vi "ORS_Samples_per_Line.vi"(2 "SPLL RF Clocks/Sweep":dbl=2560.0, 3 "Buffer_factor":i32=1, 4 "f_FDML":dbl=100000.0, 5 "General state cluster":T5={"millisecond timer value"=0, "PreviewSetNumberOfLines"=512, "Data source"=enum."AlazarTec", "DLL path"=path "M:/Optores_MHzImaging/WWImgDLL/wwimg-x86_64.dll", "n_threads"=1, "selected A-scan"={[], "cut_data"=[]}, "FDML freq"=100000.0, "Sample Rate"=500000000.0, "n_channel"=1, "Peak samp pos\n1mm (Michels)"=143, "Buffer factor"=1, "At9462Acq"={"sample_rate"=0, "clock source"=1}, "At9462Trig"={"trig_source"=enum."Ext", "trig_slope"=0, "trig_level"=0, "trig_timeout_ms"=0}, "At9462Ch1"={"coupling"=0, "range"=0, "impedance"=0}, "At9462Ch2"={"coupling"=0, "range"=0, "impedance"=0}, "At9462 # samples"=2560, "image height (crop)"=512, "B scan offset (sps)"=0.0, "window"=0, "OCT data dir"=path "", "2d file name"="", "3d file name"="", "# lines 2d"=1024, "Description"="", "Various parameters"="", "# linesPreview/jpg"=512, "# lines 3d"=512, "Y center 3d"=0.0, "Y span 3d"=0.0, "Galvo params only for file storage"={"n_lines"=400, "n_frames"=100, "force to zero"=TRUE, "Triggers_per_sweep"=1.0, "X center"=0.0, "X span"=5.6, "Y center"=0.0, "Y span"=0.0, "flyb.lines"=100, "n_triggers"=1, "mode"=3, "offset"=0.0, "galvo phase"=-15, "span factor"=0.0, "Custom trig."={"n_frames to c. trig"=0, "custom trig length (frames)"=0, "n_frames between c. trig"=0, "n_c. trig"=0}, "frames_per_pos"=5, "n_dataset"=1, "flyback fr"=0}, "Per Channel Params"=[{"AcqCursorList"=[{"Name"="img start", "Color"=16776960, "Style"=8, "Point Style"=13, "Name Visible"=FALSE, "Allow Drag"=TRUE, "Cursor Mode"=0, "Plot"=0, "Index"=0, "Position"={"X"=0.0, "Y"=50000.0}, "X Scale"=0, "Y Scale"=0, "Watch Plots"=[], "Watch All Plots"=FALSE, "Plot Area"=0, "Label Offset"={"X"=0.0, "Y"=5693.779904306226}}, {"Name"="img stop", "Color"=16776960, "Style"=8, "Point Style"=13, "Name Visible"=FALSE, "Allow Drag"=TRUE, "Cursor Mode"=0, "Plot"=0, "Index"=0, "Position"={"X"=2559.0, "Y"=50000.0}, "X Scale"=0, "Y Scale"=0, "Watch Plots"=[], "Watch All Plots"=FALSE, "Plot Area"=0, "Label Offset"={"X"=0.0, "Y"=6076.5550239234435}}, {"Name"="recal start", "Color"=16711680, "Style"=8, "Point Style"=13, "Name Visible"=FALSE, "Allow Drag"=TRUE, "Cursor Mode"=0, "Plot"=0, "Index"=0, "Position"={"X"=0.0, "Y"=50000.0}, "X Scale"=0, "Y Scale"=0, "Watch Plots"=[], "Watch All Plots"=FALSE, "Plot Area"=0, "Label Offset"={"X"=0.0, "Y"=6076.5550239234435}}, {"Name"="recal stop", "Color"=16711680, "Style"=8, "Point Style"=13, "Name Visible"=FALSE, "Allow Drag"=TRUE, "Cursor Mode"=0, "Plot"=0, "Index"=0, "Position"={"X"=2559.0, "Y"=50000.0}, "X Scale"=0, "Y Scale"=0, "Watch Plots"=[], "Watch All Plots"=FALSE, "Plot Area"=0, "Label Offset"={"X"=0.0, "Y"=6459.330143540676}}], "RecalFringePhaseFit_Inv"=array1x2560[2560 elements], "RawDualBackgroundArray"=array100x2560[256000 elements], "RawSingleBackgroundArray"=[], "RawRecalFringeArray"=array1x2560[2560 elements], "RecalFringePhaseFit"=array1x2560[2560 elements], "SingleBackground"=[], "DualBackground"=array[2560 elements], "image crop start"=0, "cut_level_low"=70.0, "cut_level_high"=110.0, "Raw1mmFringeArray"=[], "img_bckg_offset"=0, "img_bckg_length"=20, "DVV"=array1x2560[2560 elements], "DVV_shift"=0}], "file version"=8} {"window" items=["Rectangle"=0, "Hanning"=1, "Hamming"=2, "Blackman-Harris"=3, "Exact Blackman"=4, "Blackman"=5, "Flat Top"=6, "4 Term B-Harris "=7, "7 Term B-Harris"=8, "Low Sidelobe"=9, "Blackman Nuttall"=11, "Triangle"=30, "Bartlett-Hanning"=31, "Bohman"=32, "Parzen"=33, "Welch"=34, "Kaiser"=60, "Dolph-Chebyshev"=61, "Gaussian"=62]; "Galvo params only for file storage"."n_dataset" min=1; "Galvo params only for file storage"."X center" format="%^_3g"; "Galvo params only for file storage"."X span" format="%^_3g"; "Galvo params only for file storage"."Y center" format="%^_3g"; "Galvo params only for file storage"."Y span" format="%^_3g"}) -> (0 "eff. FDML frequency":dbl=100000.0, 1 "samples per line":dbl)   [LabVIEW 2014]
uses:
  <vilib>/Analysis/4window.llb/windowTd.ctl
  Typedefs/ORS_Galvo_params.ctl
  Typedefs/ORS_Per_Ch_params.ctl
  <vilib>/Utility/miscctls.llb/LVCursorListTypeDef.ctl
  <vilib>/Analysis/NI_AALPro.lvlib
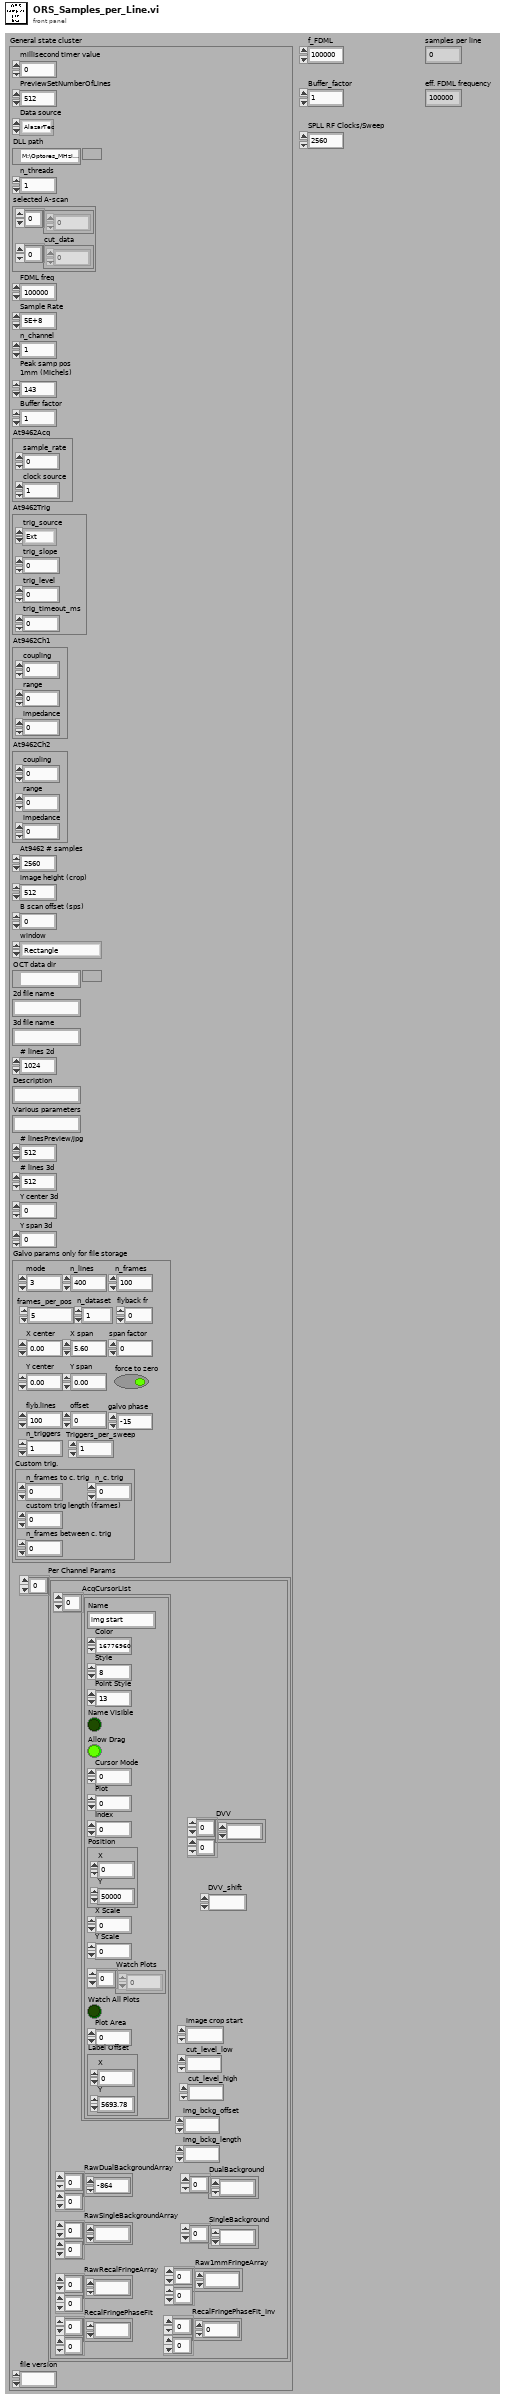
[diagram p1: front panel]
types:
  T1 = typedef "NI_AALPro.lvlib/windowTd.ctl" = u32
  T2 = typedef "ORS_Galvo_params.ctl" = cluster{"n_lines":i32, "n_frames":i32, "force to zero":bool, "Triggers_per_sweep":dbl, "X center":dbl, "X span":dbl, "Y center":dbl, "Y span":dbl, "flyb.lines":i32, "n_triggers":i32, "mode":i32, "offset":dbl, "galvo phase":i32, "span factor":dbl, "Custom trig.":cluster{"n_frames to c. trig":i32, "custom trig length (frames)":i32, "n_frames between c. trig":i32, "n_c. trig":i32}, "frames_per_pos":i32, "n_dataset":u32, "flyback fr":u16}
  T3 = typedef "ORS_Per_Ch_params.ctl" = cluster{"AcqCursorList":T4, "RecalFringePhaseFit_Inv":dbl[][], "RawDualBackgroundArray":i16[][], "RawSingleBackgroundArray":i16[][], "RawRecalFringeArray":i16[][], "RecalFringePhaseFit":dbl[][], "SingleBackground":i16[], "DualBackground":i16[], "image crop start":i32, "cut_level_low":dbl, "cut_level_high":dbl, "Raw1mmFringeArray":i16[][], "img_bckg_offset":i32, "img_bckg_length":i32, "DVV":i16[][], "DVV_shift":i32}[]
  T4 = typedef "LVCursorListTypeDef.ctl" = cluster{"Name":string, "Color":u32, "Style":u8, "Point Style":u8, "Name Visible":bool, "Allow Drag":bool, "Cursor Mode":u32, "Plot":i32, "Index":i32, "Position":cluster{"X":dbl, "Y":dbl}, "X Scale":u32, "Y Scale":u32, "Watch Plots":i32[], "Watch All Plots":bool, "Plot Area":i32, "Label Offset":cluster{"X":dbl, "Y":dbl}}[]
  T5 = cluster{"millisecond timer value":u32, "PreviewSetNumberOfLines":i32, "Data source":enum32{"AlazarTec"}, "DLL path":path, "n_threads":i32, "selected A-scan":cluster{dbl[], "cut_data":dbl[]}, "FDML freq":dbl, "Sample Rate":dbl, "n_channel":i32, "Peak samp pos\n1mm (Michels)":i32, "Buffer factor":i32, "At9462Acq":cluster{"sample_rate":u32, "clock source":u32}, "At9462Trig":cluster{"trig_source":enum16{"Ext", "A", "B", "Off"}, "trig_slope":i32, "trig_level":i32, "trig_timeout_ms":i32}, "At9462Ch1":cluster{"coupling":i32, "range":i32, "impedance":i32}, "At9462Ch2":cluster{"coupling":i32, "range":i32, "impedance":i32}, "At9462 # samples":u32, "image height (crop)":i32, "B scan offset (sps)":dbl, "window":T1, "OCT data dir":path, "2d file name":string, "3d file name":string, "# lines 2d":i32, "Description":string, "Various parameters":string, "# linesPreview/jpg":i32, "# lines 3d":i32, "Y center 3d":dbl, "Y span 3d":dbl, "Galvo params only for file storage":T2, "Per Channel Params":T3, "file version":u32}
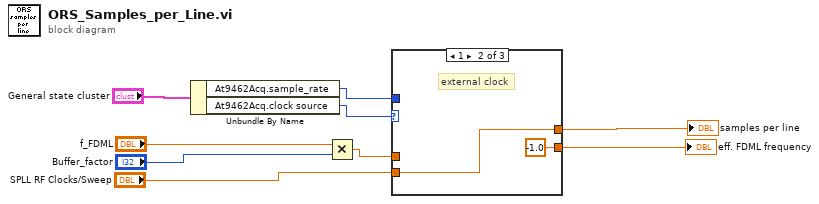
[diagram p0: block diagram]
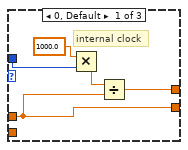
[diagram p2: hidden frame]
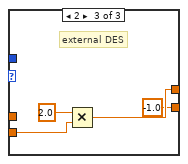
[diagram p3: hidden frame]
diagram:
  n1 = Unbundle By Name("General state cluster") -> ("At9462Acq.sample_rate"=w4:u32, "At9462Acq.clock source"=w7:u32)
  n2 = Multiply(x="f_FDML", y="Buffer_factor") -> (x*y=w3:dbl)
  n3 = case shown="1" w7 {
    tunnel: w3 -> [w10 _ _]
    tunnel: w4 -> [w14 _ _]
    tunnel: [w11 w16 w18] -> w6
    tunnel: "SPLL RF Clocks/Sweep" -> [_ w16 w20]
    tunnel: [w10 -1.0 -1.0] -> w9
    frame 0, Default {
      # "internal clock"
      n4 = Multiply(x=1000.0, y=w14) -> (x*y=w12:dbl)
      n5 = Divide(x=w12, y=w10) -> (x/y=w11:dbl)
    }
    frame 1 {
      # "external clock"
    }
    frame 2 {
      # "external DES"
      n6 = Multiply(x=2.0, y=w20) -> (x*y=w18:dbl)
    }
  }
  "eff. FDML frequency" <- w9
  "samples per line" <- w6
